vi "UARTDATA.vi"() -> ()   [LabVIEW 2021]
uses:
  <vilib>/Instr/_visa.llb/VISA Configure Serial Port (Instr).vi
panel:
  in  "Tab Control":T1(tab)
  in  "VISA resource name":refnum<visa-resource-name>
  out "READ BUFFER":string
  out "DATA":string
  out "DATA SEN":string[](array[string])
  out "BTNC":bool
  out "BTNB":bool
  out "BTNA":bool caption="Boolean"
  in  "stop":bool
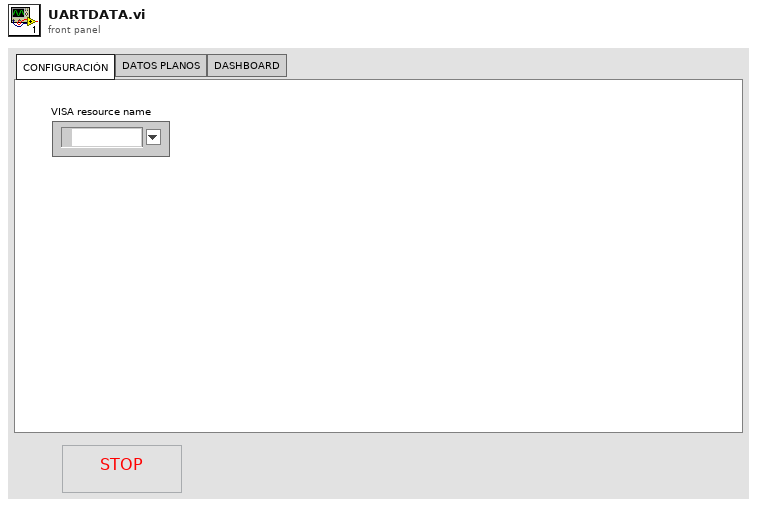
[diagram p1: front panel]
types:
  T1 = enum32{"CONFIGURACIÓN", "DATOS PLANOS", "DASHBOARD"}
  T2 = enum16{"ESPERAR DATA", "LEER DATA", "INTERPRETAR DATA", "VISUALIZAR DATA"}
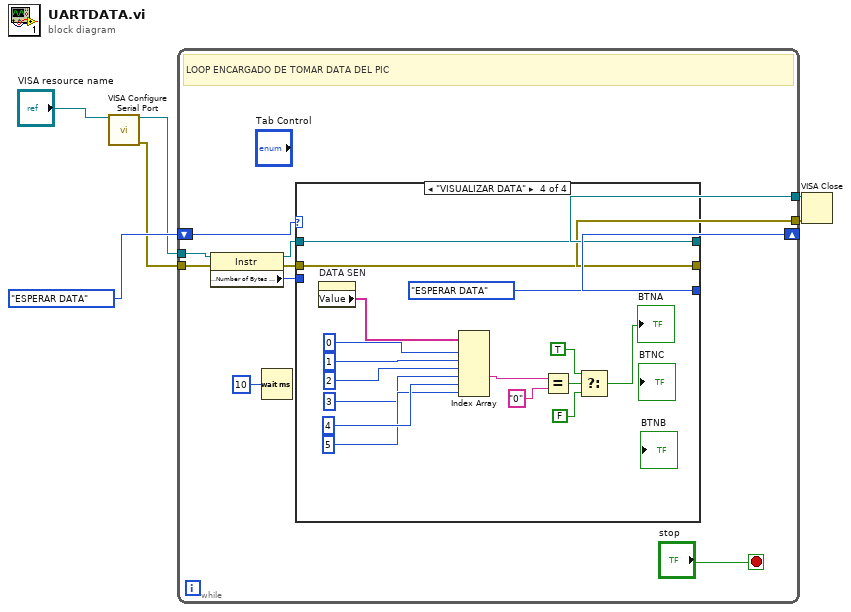
[diagram p0: block diagram]
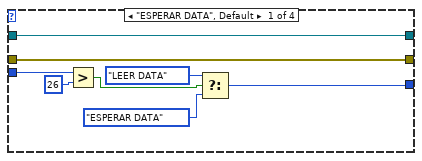
[diagram p2: hidden frame]
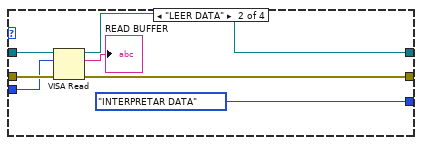
[diagram p3: hidden frame]
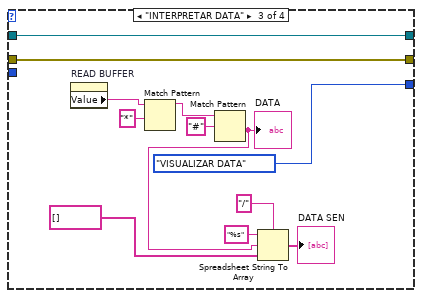
[diagram p4: hidden frame]
diagram:
  n1 = call-poly "VISA Configure Serial Port"("VISA resource name"="VISA resource name") -> ("VISA resource name out"=w4:refnum<visa-resource-name>, "error out"=w3:errorcluster)  [unwired: 13 in]
  n2 = while {
    shift-right: [w11] -> _
    shift-left: T2."ESPERAR DATA" -> [w15]
    tunnel: w4 -> [w14]
    tunnel: w3 -> [w13]
    tunnel: [w8] -> w2
    tunnel: [w7] -> w1
    stop <- "stop" stop-if-true
    # "LOOP ENCARGADO DE TOMAR DATA DEL PIC"
    n3 = property class="Instr"(reference=w14, error in=w13) -> (reference out=w10:refnum<visa-resource-name>, error out=w9:errorcluster, "Serial Settings:Number of Bytes at Serial Port"=w12:u32)
    n4 = Wait (ms)(milliseconds to wait=u32 10) -> ()  [unwired: 1 out]
    n5 = case shown="\"VISUALIZAR DATA\"" w15 {
      tunnel: w12 -> [w25 w30 _ _]
      tunnel: [w20 T2."INTERPRETAR DATA" T2."VISUALIZAR DATA" T2."ESPERAR DATA"] -> w11
      tunnel: w10 -> [w19 w32 w43 w59]
      tunnel: w9 -> [w18 w31 w42 w58]
      tunnel: [w19 w27 w43 w59] -> w8
      tunnel: [w18 w26 w42 w58] -> w7
      frame "ESPERAR DATA", Default {
        n6 = Greater?(x=w25, y=u32 26) -> (0:w23:bool)
        n7 = Select(t=T2."LEER DATA", s=w23, f=T2."ESPERAR DATA") -> (s? t:f=w20:T2)
      }
      frame "LEER DATA" {
        n8 = VISA Read(VISA resource name=w32, byte count=w30, error in (no error)=w31) -> (VISA resource name out=w27:refnum<visa-resource-name>, read buffer=→"READ BUFFER":string, error out=w26:errorcluster)  [unwired: 1 out]
      }
      frame "INTERPRETAR DATA" {
        n9 = property on="READ BUFFER" class="Str"() -> ("Value"=w41:string)  [unwired: 2 in, 2 out]
        n10 = Match Pattern(string=w41, regular expression="*") -> (before substring=w39:string)  [unwired: 1 in, 3 out]
        n11 = Match Pattern(string=w39, regular expression="#") -> (after substring=w35:string)  [unwired: 1 in, 3 out]
        "DATA" <- w35
        n12 = Spreadsheet String To Array(delimiter (Tab)="/", format string="%s", spreadsheet string=w35, array type (2D Dbl)=string[] []) -> (array=→"DATA SEN":string[])
      }
      frame "VISUALIZAR DATA" {
        n13 = property on="DATA SEN" class="Arr (strict)"() -> ("Value"=w57:string[])  [unwired: 2 in, 2 out]
        n14 = Index Array(array=w57, index #1=0 ("index"), index #2=1 ("index"), index #3=2 ("index"), index #4=3 ("index"), index #5=4 ("index"), index #6=5 ("index")) -> (element #4=w50:string)  [unwired: 5 out]
        n15 = Equal?(x=w50, y="0") -> (x = y?=w48:bool)
        n16 = Select(t=TRUE, s=w48, f=FALSE) -> (s? t:f=→"BTNA":bool)
      }
    }
  }
  n17 = VISA Close(VISA resource name=w2, error in (no error)=w1) -> ()  [unwired: 1 out]
